vi "Read ExtractImages.vi"(8 "error in (no error)":errorcluster, 11 "Vision in":refnum<class "Vision.lvclass">) -> (0 "error out":errorcluster, 2 "ExtractImages":T1[](array[typedef]), 3 "Vision out":refnum<class "Vision.lvclass">)   [LabVIEW 2021, in "Vision.lvlib" / "Vision.lvclass"]
uses:
  Vision.lvclass
  <vilib>/vision/Image Controls.llb/IMAQ Image.ctl
  Vision.lvclass/Vision.ctl
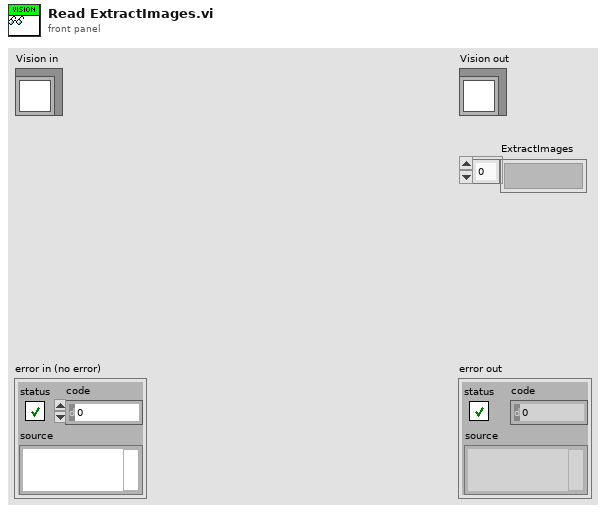
[diagram p1: front panel]
types:
  T1 = typedef "IMAQ Image.ctl" = refnum<image>
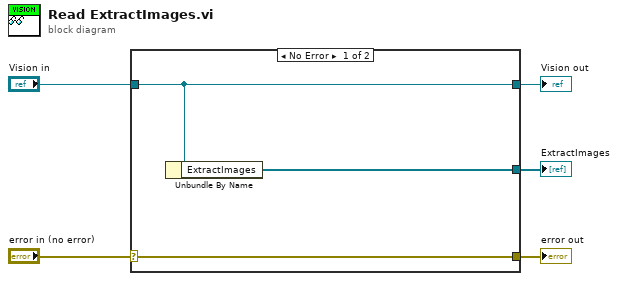
[diagram p0: block diagram]
diagram:
  n1 = case shown="No Error" "error in (no error)" {
    selector: "error in (no error)" -> [w8 w9]
    tunnel: [w8 w9] -> w4
    tunnel: [w7 w10] -> w2
    tunnel: "Vision in" -> [w7 w10]
    tunnel: [w6 _] -> w1
    frame No Error {
      n2 = Unbundle By Name(w7) -> ("ExtractImages"=w6:T1[])
    }
    frame Error {
    }
  }
  "error out" <- w4
  "Vision out" <- w2
  "ExtractImages" <- w1
